vi "Create Directory Structure.vi"(4 "error in":errorcluster, 7 "Path":path) -> (0 "error out":errorcluster, 3 "dup Path":path)   [LabVIEW 2015]
doc: "Create Directory Structure.vi version 1.0\nThis VI takes an input path and verifies that the path already exists. If it does not, it attempts to create the path, creating as many nested directories as necessary starting with the highest level directory that already existed.\n\nOriginal Code by David Thomson Original Code Consulting May, 2003\n www.originalcode.com\n\nThis VI is available as freeware for use by the LabVIEW community, with the sole condition being that the attribution to the author be left intact in this documentation."
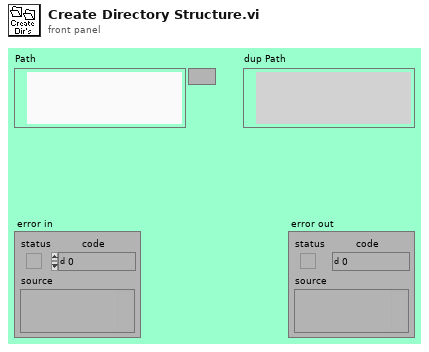
[diagram p1: front panel]
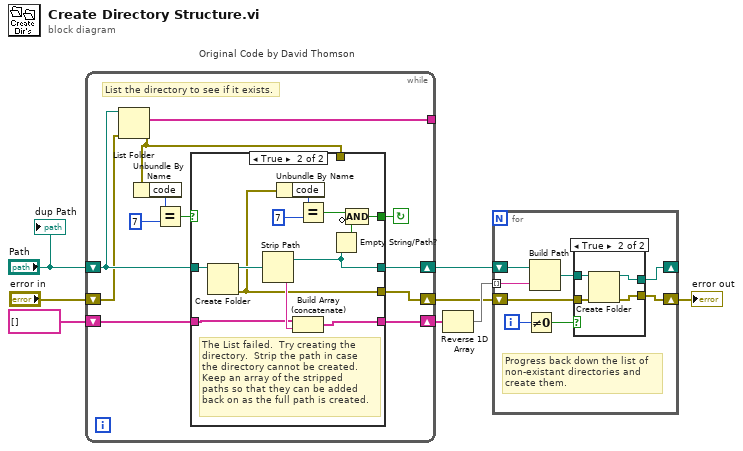
[diagram p0: block diagram]
diagram:
  n1 = while "Original Code by David Thomson" {
    tunnel: [w19] -> _
    shift-right: [w18] -> w5
    shift-left: "Path" -> [w20]
    shift-right: [w13] -> w7
    shift-left: string[] [] -> [w12]
    shift-right: [w9] -> w2
    shift-left: "error in" -> [w11]
    stop <- w17 continue-if-true
    # "List the directory to see if it exists."
    n2 = List Folder(path=w20, error in=w11) -> (filenames=w19:string[], error out=w10:errorcluster)  [unwired: 4 out]
    n3 = Unbundle By Name(w10) -> ("code"=w16:i32)
    n4 = Equal?(x=w16, y=7) -> (x = y?=w14:bool)
    n5 = case shown="True" w14 {
      selector: w14 -> [w24 _]
      tunnel: w20 -> [w23 w36]
      tunnel: [w23 w33] -> w18
      tunnel: [w24 w34] -> w17
      tunnel: [w22 w25] -> w9
      tunnel: w10 -> [w22 _]
      tunnel: [w21 w29] -> w13
      tunnel: w12 -> [w21 w30]
      frame False {
        # "The directory was found.\nStop parsing up the\ndirectory structure."
      }
      frame True {
        # "The List failed.  Try creating the\ndirectory.  Strip the path in case\nthe directory cannot be created.\nKeep an array of the stripped\npaths so that they can be added\nback on as the full path is created."
        n6 = Create Folder(path (use dialog)=w36) -> (created path=w35:path, error out=w25:errorcluster)  [unwired: 1 in, 2 out]
        n7 = Strip Path(path=w35) -> (stripped path=w33:path, name=w31:string)
        n8 = Unbundle By Name(w25) -> ("code"=w27:i32)
        n9 = Build Array (concatenate)(w30, w31) -> (w29:string[])
        n10 = Equal?(x=w27, y=7) -> (x = y?=w26:bool)
        n11 = Empty String/Path?(string/path=w33) -> (empty?=w32:bool)
        n12 = Compound Arithmetic op=AND(w26, invert w32) -> (w34:bool)
      }
    }
  }
  n13 = Reverse 1D Array(array=w7) -> (reversed array=w4:string[])
  n14 = for {
    tunnel: w4 -> [w43] mode=indexing
    shift-right: [w40] -> w6
    shift-left: w2 -> [w41]
    shift-right: [w39] -> _
    shift-left: w5 -> [w44]
    i -> [w37]
    # "Progress back down the list of\nnon-existant directories and\ncreate them."
    n15 = Not Equal To 0?(x=w37) -> (x != 0?=w38:bool)
    n16 = Build Path(base path=w44, name or relative path=w43) -> (appended path=w42:path)
    n17 = case shown="True" w38 {
      tunnel: w42 -> [w46 w50]
      tunnel: w41 -> [w45 w49]
      tunnel: [w45 w48] -> w40
      tunnel: [w46 w47] -> w39
      frame False {
      }
      frame True {
        n18 = Create Folder(path (use dialog)=w50, error in=w49) -> (created path=w47:path, error out=w48:errorcluster)  [unwired: 2 out]
      }
    }
  }
  "error out" <- w6
  "dup Path" <- "Path"
